vi "SocialDoor.vi"(9 "Override":bool, 10 "Interaction time":u32) -> ()   [LabVIEW 2021]
uses:
  <vilib>/DAQmx/write.llb/DAQmx Write (Digital Bool 1Line 1Point).vi
  <vilib>/DAQmx/create/channels.llb/DAQmx Create Channel (DO-Digital Output).vi
  <vilib>/DAQmx/miscellaneous.llb/DAQmx Fill In Error Info.vi
  Global_BeamBreaks.vi
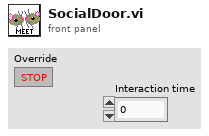
[diagram p1: front panel]
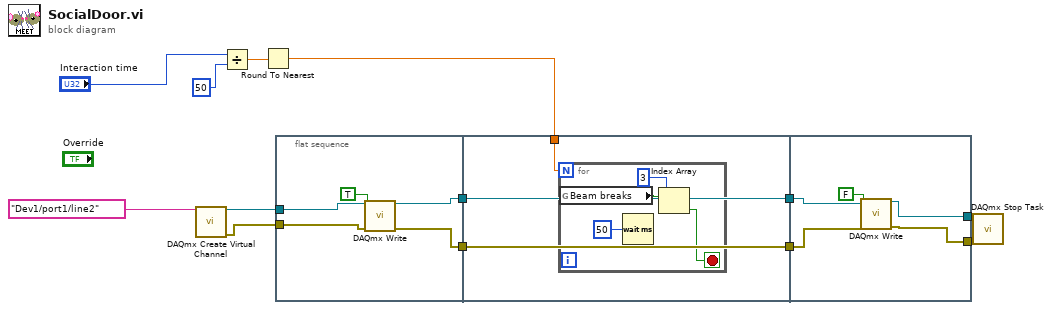
[diagram p0: block diagram]
diagram:
  n1 = call-poly <vilib>:"DAQmx Create Virtual Channel.vi"("lines"=tag "Dev1/port1/line2") -> ("task out"=w13:refnum<k21>, "error out"=w10:errorcluster)  [unwired: 13 in]
  n2 = Divide(x="Interaction time", y=u32 50) -> (x/y=w2:dbl)
  n3 = Round To Nearest(number=w2) -> (nearest integer value=w1:dbl)
  n4 = flat-sequence {
    tunnel: w13 -> [w18]
    tunnel: [w17] -> w11
    tunnel: w10 -> [w16]
    tunnel: [w15] -> w8
    tunnel: [w21] -> w12
    tunnel: w11 -> [w21]
    tunnel: [w20] -> w9
    tunnel: w8 -> [w20]
    tunnel: w1 -> [w19]
    tunnel: w12 -> [w30]
    tunnel: w9 -> [w29]
    tunnel: [w28] -> w7
    tunnel: [w27] -> w6
    frame #0 {
      n5 = call-poly <vilib>:"DAQmx Write.vi"("task/channels in"=w18, "data"=TRUE, "error in"=w16) -> ("task out"=w17:refnum<k21>, "error out"=w15:errorcluster)  [unwired: 10 in, 1 out]
    }
    frame #1 {
      n6 = for {
        N: w19 -> [_]
        stop <- w22 stop-if-true
        n7 = global read "Global_BeamBreaks.vi" "Beam breaks"() -> (w24:bool[])
        n8 = Wait (ms)(milliseconds to wait=u32 50) -> ()  [unwired: 1 out]
        n9 = Index Array(array=w24, index=3) -> (element=w22:bool)
      }
    }
    frame #2 {
      n10 = call-poly <vilib>:"DAQmx Write.vi"("task/channels in"=w30, "data"=FALSE, "error in"=w29) -> ("task out"=w28:refnum<k21>, "error out"=w27:errorcluster)  [unwired: 10 in, 1 out]
    }
  }
  n11 = call <vilib>:"DAQmx Stop Task.vi"("task/channels in"=w7, "error in"=w6) -> ()  [unwired: 12 in, 2 out]
